vi "Manniquin Control.vi"(7 "Position":T1, 8 "error in (no error)":errorcluster, 11 "Queue in":refnum<queue>) -> (0 "error out":errorcluster, 3 "Queue out":refnum<queue>)   [LabVIEW 2020]
uses:
  Message Queue/Message Cluster.ctl
  Mannequin and Gas Position.ctl
  Message Queue/Enqueue Message (Single).vi
  Message Queue/Message Queue.lvlib
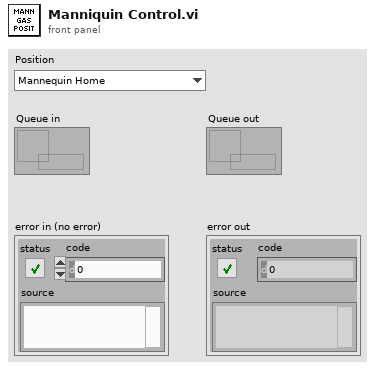
[diagram p1: front panel]
types:
  T1 = typedef "Mannequin and Gas Position.ctl" = enum16{"Mannequin Home", "Mannequin Work", "Gas Can Home", "Gas Can Work"}
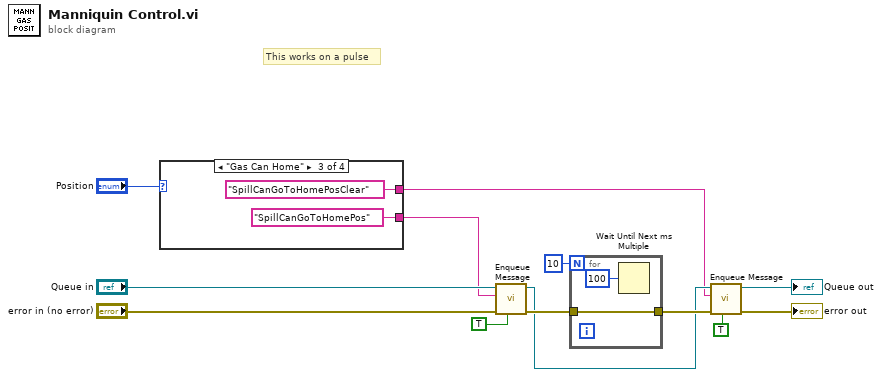
[diagram p0: block diagram]
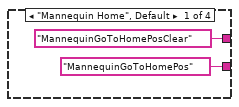
[diagram p2: hidden frame]
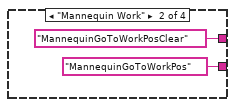
[diagram p3: hidden frame]
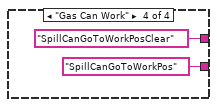
[diagram p4: hidden frame]
diagram:
  # "This works on a pulse"
  n1 = case shown="\"Gas Can Home\"" "Position" {
    tunnel: ["MannequinGoToHomePos" ("Message") "MannequinGoToWorkPos" ("Message") "SpillCanGoToHomePos" ("Message") "SpillCanGoToWorkPos" ("Message")] -> w5
    tunnel: ["MannequinGoToHomePosClear" ("Message") "MannequinGoToWorkPosClear" ("Message") "SpillCanGoToHomePosClear" ("Message") "SpillCanGoToWorkPosClear" ("Message")] -> w4
    frame "Mannequin Home", Default {
    }
    frame "Mannequin Work" {
    }
    frame "Gas Can Home" {
    }
    frame "Gas Can Work" {
    }
  }
  n2 = call-poly "Enqueue Message.vi"("Priority Message? (F)"=TRUE, "error in (no error)"="error in (no error)", "Message"=w5, "Message Queue"="Queue in") -> ("error out"=w11:errorcluster, "dup Message Queue"=w7:refnum<queue>)  [unwired: 6 in]
  n3 = for {
    N: 10 -> [_]
    tunnel: w11 -> [w22]
    tunnel: [w22] -> w12
    n4 = Wait Until Next ms Multiple(millisecond multiple=u32 100) -> ()  [unwired: 1 out]
  }
  n5 = call-poly "Enqueue Message.vi"("Priority Message? (F)"=TRUE, "error in (no error)"=w12, "Message"=w4, "Message Queue"=w7) -> ("error out"=→"error out":errorcluster, "dup Message Queue"=→"Queue out":refnum<queue>)  [unwired: 6 in]
